vi "ma_SML Window Parameters.vi"(0 "window":u16(ring) items=["Rectangle"=0, "Hanning"=1, "Hamming"=2, "Blackman-Harris"=3, "Exact Blackman"=4, "Blackman"=5, "Flat Top"=6, "4 Term B-Harris "=7, "7 Term B-Harris"=8, "Low Sidelobe"=9, "Blackman Nuttall"=11, "Triangle"=30, "Bartlett-Hanning"=31, "Bohman"=32, "Parzen"=33, "Welch"=34, "Kaiser"=60, "Dolph-Chebyshev"=61, "Gaussian"=62]) -> (1 "coherent gain":dbl format="%.2f", 2 "ENBW":dbl format="%.2f", 3 "3dB BW":dbl format="%.2f", 4 "6dB BW":dbl format="%.2f")   [LabVIEW 2020, in "NI_MAPro.lvlib"]
uses:
  NI_MAPro.lvlib
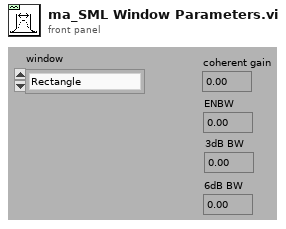
[diagram p1: front panel]
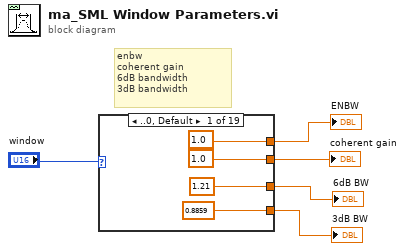
[diagram p0: block diagram]
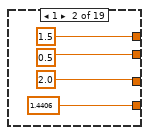
[diagram p2: hidden frame]
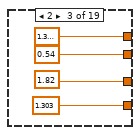
[diagram p3: hidden frame]
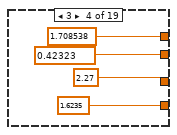
[diagram p4: hidden frame]
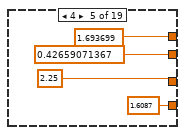
[diagram p5: hidden frame]
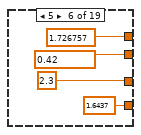
[diagram p6: hidden frame]
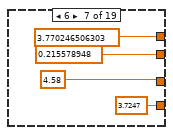
[diagram p7: hidden frame]
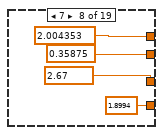
[diagram p8: hidden frame]
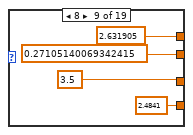
[diagram p9: hidden frame]
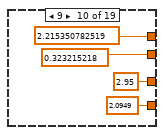
[diagram p10: hidden frame]
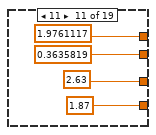
[diagram p11: hidden frame]
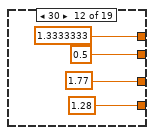
[diagram p12: hidden frame]
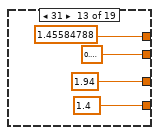
[diagram p13: hidden frame]
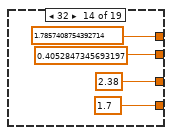
[diagram p14: hidden frame]
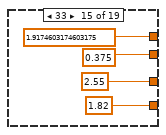
[diagram p15: hidden frame]
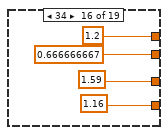
[diagram p16: hidden frame]
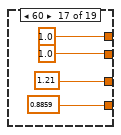
[diagram p17: hidden frame]
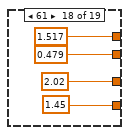
[diagram p18: hidden frame]
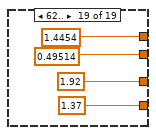
[diagram p19: hidden frame]
diagram:
  # "enbw\ncoherent gain\n6dB bandwidth\n3dB bandwidth"
  n1 = case shown="..0, Default" "window" {
    tunnel: [1.0 0.5 0.54 0.42323 0.42659071367 0.42 0.215578948 0.35875 0.27105140069342415 0.323215218 0.3635819 ("coherent gain") 0.5 ("coherent gain") 0.49999999999998385 ("coherent gain") 0.4052847345693197 ("coherent gain") 0.375 ("coherent gain") 0.666666667 ("coherent gain") 1.0 ("coherent gain") 0.479 ("coherent gain") 0.49514 ("coherent gain")] -> w4
    tunnel: [1.0 1.5 1.362826 1.708538 1.693699 1.726757 3.770246506303 2.004353 2.631905 2.215350782519 1.9761117 ("eq noise BW") 1.3333333 ("eq noise BW") 1.45584788 ("eq noise BW") 1.7857408754392714 ("eq noise BW") 1.9174603174603175 ("eq noise BW") 1.2 ("eq noise BW") 1.0 ("eq noise BW") 1.517 ("eq noise BW") 1.4454 ("eq noise BW")] -> w5
    tunnel: [1.21 2.0 1.82 2.27 2.25 2.3 4.58 2.67 3.5 2.95 2.63 1.77 1.94 2.38 2.55 1.59 1.21 2.02 1.92] -> w3
    tunnel: [0.8859 1.4406 1.303 1.6235 1.6087 1.6437 3.7247 1.8994 2.4841 2.0949 1.87 1.28 1.4 1.7 1.82 1.16 0.8859 1.45 1.37] -> w1
    frame ..0, Default {
    }
    frame 1 {
    }
    frame 2 {
    }
    frame 3 {
    }
    frame 4 {
    }
    frame 5 {
    }
    frame 6 {
    }
    frame 7 {
    }
    frame 8 {
    }
    frame 9 {
    }
    frame 11 {
    }
    frame 30 {
    }
    frame 31 {
    }
    frame 32 {
    }
    frame 33 {
    }
    frame 34 {
    }
    frame 60 {
    }
    frame 61 {
    }
    frame 62.. {
    }
  }
  "ENBW" <- w5
  "coherent gain" <- w4
  "6dB BW" <- w3
  "3dB BW" <- w1
